vi "NIClustering_Kmeans.vi"(5 "Enum":enum16{"KLD", "Euclidean"}(ring), 7 "type":enum16{"Generate", "Input"}(ring), 9 "Centroids in":dbl[][](array[numeric]), 10 "Classes":i32=2, 11 "Data":T1=[[30.0, 100.0, 20.0], [50.0, 60.0, 40.0]]) -> (0 "distance":dbl[][](array[numeric]), 2 "Centroids":T1, 3 "Results":i32[](array[numeric]))   [LabVIEW 2014]
uses:
  <vilib>/Analysis/Matrix/Datatypes/RealMatrix.ctl
  <vilib>/Analysis/_algsub.llb/Real Matrix Norm.vi
  <vilib>/Analysis/7linalg.llb/Real Transpose Matrix.vi
  <vilib>/addons/Clustering/Algorithms/Clustering.llb/NIClustering_Global.vi
  <vilib>/Analysis/NI_AALPro.lvlib
  <vilib>/Analysis/Matrix/NI_Matrix.lvlib
panel:
  out "N":i32
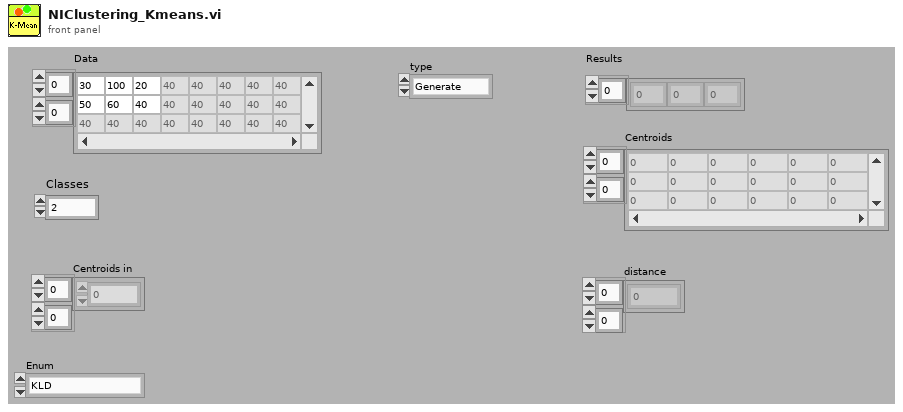
[diagram p1: front panel]
types:
  T1 = typedef "NI_Matrix.lvlib/RealMatrix.ctl" = dbl[][]
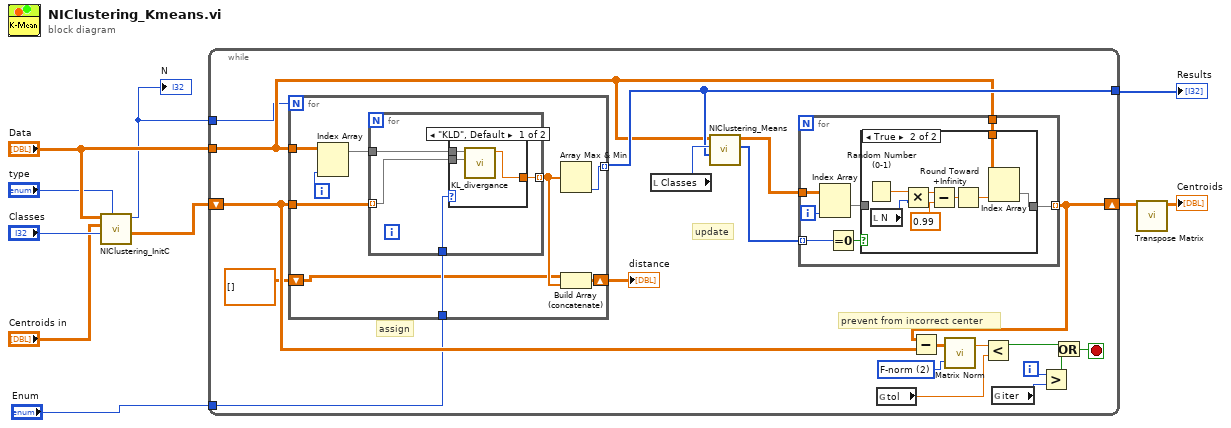
[diagram p0: block diagram]
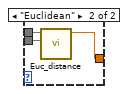
[diagram p3: hidden frame]
diagram:
  n1 = call <vilib>:"NIClustering_InitC.vi"("type"="type", "Classes"="Classes", "Centroids in"="Centroids in", "Data"="Data") -> ("Centroids"=w6:dbl[][], "Sample number"=w4:i32)  [unwired: 6 in]
  "N" <- w4
  n2 = while {
    shift-right: [w24] -> w8
    shift-left: w6 -> [w30]
    tunnel: "Data" -> [w17]
    tunnel: [w20] -> w7
    tunnel: w4 -> [w16]
    tunnel: "Enum" -> [w13]
    i -> [w26]
    stop <- w25 stop-if-true
    w28 = 2 items=["2-norm", "1-norm", "F-norm", "Inf-norm"] ("norm type")
    # "prevent from incorrect center"
    # "update"
    # "assign"
    n3 = for {
      N: w16 -> [_]
      tunnel: w30 -> [w55]
      tunnel: [w54] -> w20 mode=indexing
      tunnel: w17 -> [w53]
      tunnel: w13 -> [w50]
      shift-right: [w48] -> w11
      shift-left: dbl[][] [] -> [w47]
      i -> [w51]
      n4 = Index Array(array=w53, index (col)=w51) -> (element=w52:dbl[])  [unwired: 1 in]
      n5 = for {
        tunnel: w55 -> [w57] mode=indexing
        tunnel: w52 -> [w58]
        tunnel: [w59] -> w49 mode=indexing
        tunnel: w50 -> [w56]
        n6 = case shown="\"KLD\", Default" w56 {
          tunnel: [w60 w65] -> w59
          tunnel: w58 -> [w62 w64]
          tunnel: w57 -> [w61 w63]
          frame "KLD", Default {
            n7 = call "KL_divergance.vi"("Centroid"=w61, "Independent\nVariable (Zi)"=w62) -> ("Euclidean\nDistance"=w60:dbl)  [unwired: 9 in]
          }
          frame "Euclidean" {
            n8 = call "Euc_distance.vi"("Centroid"=w63, "Values (row = members, \ncolumn = sample Num)"=w64) -> ("Euclidean\nDistance"=w65:dbl)  [unwired: 9 in]
          }
        }
      }
      n9 = Array Max & Min(array=w49) -> (min index (indices)=w54:i32)  [unwired: 3 out]
      n10 = Build Array (concatenate)(w47, w49) -> (w48:dbl[][])
    }
    "distance" <- w11
    n11 = local read "Classes"() -> (w21:i32)
    n12 = call <vilib>:"NIClustering_Means.vi"("Results"=w20, "Classes"=w21, "Data"=w17) -> ("Numbers"=w19:i32[], "Means"=w18:T1)  [unwired: 7 in]
    n13 = for {
      tunnel: w19 -> [w35] mode=indexing
      tunnel: w17 -> [w37]
      tunnel: w18 -> [w33]
      tunnel: [w36] -> w24 mode=indexing
      i -> [w32]
      n14 = Index Array(array=w33, index (col)=w32) -> (element=w31:dbl[])  [unwired: 1 in]
      n15 = Equal To 0?(x=w35) -> (x = 0?=w34:bool)
      n16 = case shown="True" w34 {
        tunnel: w31 -> [w38 _]
        tunnel: w37 -> [_ w46]
        tunnel: [w38 w40] -> w36
        frame False {
        }
        frame True {
          n17 = Random Number (0-1)() -> (number: 0 to 1=w43:dbl)
          n18 = local read "N"() -> (w41:i32)
          n19 = Multiply(x=w43, y=w41) -> (x*y=w45:dbl)
          n20 = Subtract(x=w45, y=0.99) -> (x-y=w44:dbl)
          n21 = Round Toward +Infinity(x=w44) -> (ceil(x): smallest int >= x=w39:dbl)
          n22 = Index Array(array=w46, index (col)=w39) -> (element=w40:dbl[])  [unwired: 1 in]
        }
      }
    }
    n23 = global read "NIClustering_Global.vi" "tol"() -> (w15:dbl)
    n24 = Subtract ("Subtract.vi")(x=w24, y=w30) -> (x-y=w29:dbl[][])
    n25 = call-poly <vilib>:"Matrix Norm.vi"("norm type"=w28, "Input Matrix"=w29) -> ("norm"=w27:dbl)  [unwired: 1 out]
    n26 = Less?(x=w27, y=w15) -> (x < y?=w23:bool)
    n27 = global read "NIClustering_Global.vi" "iter"() -> (w14:i32)
    n28 = Greater?(x=w26, y=w14) -> (0:w22:bool)
    n29 = Or(x=w23, y=w22) -> (x .or. y?=w25:bool)
  }
  "Results" <- w7
  n30 = call-poly <vilib>:"Transpose Matrix.vi"("Input Matrix"=w8) -> ("Matrix Transpose"=→"Centroids":T1)  [unwired: 9 in, 1 out]
